vi "Add ECAT Slave.vi"(8 "error in (no error)":errorcluster, 11 "ECAT Master Ref in":T1 format="%.0x") -> (0 "error out":errorcluster, 3 "ECAT Master Ref out":T1 format="%.0x")   [LabVIEW 2016, in "Scan Engine Custom Device.lvlib"]
uses:
  Scan Engine Custom Device.lvlib
  <vilib>/NI Veristand/Custom Device API/Custom Device API.lvlib
  Globals/Scan Engine GUIDs.vi
  Globals/Property Strings.vi
  Type Defs/NI ECAT Slaves.ctl
  <vilib>/NI Veristand/Custom Device API/Custom Device Item Ref.ctl
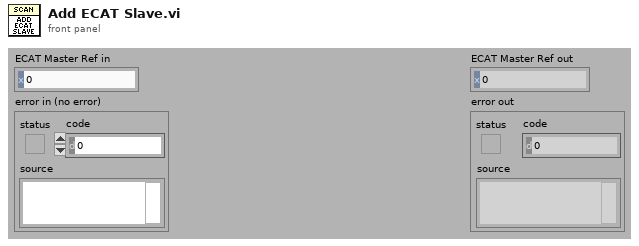
[diagram p1: front panel]
types:
  T1 = typedef "Custom Device API.lvlib/Custom Device Item Ref.ctl" = u64
  T2 = typedef "Scan Engine Custom Device.lvlib/NI ECAT Slaves.ctl" = enum16{"Default", "NI 9144"}
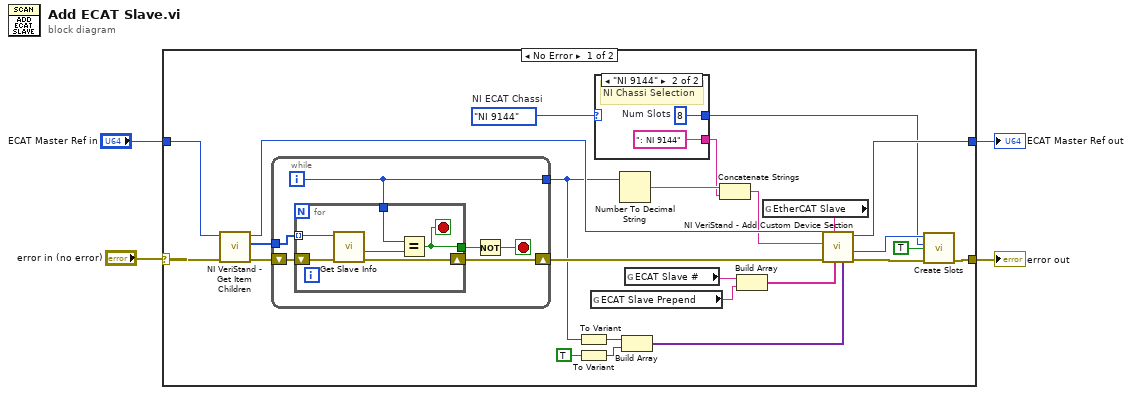
[diagram p0: block diagram]
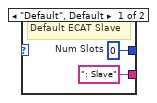
[diagram p2: hidden frame]
diagram:
  n1 = case shown="No Error" "error in (no error)" {
    selector: "error in (no error)" -> [w29 w47]
    tunnel: [w16 w47] -> w3
    tunnel: "ECAT Master Ref in" -> [w28 w46]
    tunnel: [w14 w46] -> w1
    frame No Error {
      w5 = NI_ECAT_Slaves."NI 9144"  # NI ECAT Chassi
      n2 = call <vilib>:"NI VeriStand - Get Item Children.vi"("error in (no error)"=w29, "Item Ref in"=w28) -> ("error out"=w27:errorcluster, "Child Refs"=w26:T1[], "Item Ref out"=w23:T1)  [unwired: 6 in, 1 out]
      n3 = while {
        shift-right: [w35] -> w24
        shift-left: w27 -> [w39]
        tunnel: w26 -> [w38]
        tunnel: [w34] -> w12
        i -> [w34]
        stop <- w36 stop-if-true
        n4 = for {
          tunnel: w38 -> [w42] mode=indexing
          shift-right: [w41] -> w35
          shift-left: w39 -> [w43]
          tunnel: w34 -> [w45]
          tunnel: [w44] -> w37
          stop <- w44 stop-if-true
          n5 = call "Get Slave Info.vi"("error in (no error)"=w43, "Item Ref in"=w42) -> ("error out"=w41:errorcluster, "Slave #"=w40:u16)  [unwired: 5 in, 3 out]
          n6 = Equal?(x=w45, y=w40) -> (x = y?=w44:bool)
        }
        n7 = Not(x=w37) -> (.not. x?=w36:bool)
      }
      n8 = To Variant(anything=w12) -> (Variant=w11:variant)
      n9 = To Variant(anything=TRUE) -> (Variant=w10:variant)
      n10 = global read "Property Strings.vi" "ECAT Slave Prepend"() -> (w13:string)
      n11 = case "Case-Struktur" shown="\"NI 9144\"" w5 {
        tunnel: [w31 w33] -> w7
        tunnel: [": Slave" ("string") ": NI 9144" ("string")] -> w6
        frame "Default", Default {
          w31 = 0  # Num Slots
          # "Default ECAT Slave"
        }
        frame "NI 9144" {
          w33 = 8  # Num Slots
          # "NI Chassi Selection"
        }
      }
      n12 = Number To Decimal String(number=w12) -> (decimal integer string=w20:string)  [unwired: 1 in]
      n13 = Build Array(w11, w10) -> (w8:variant[])
      n14 = global read "Property Strings.vi" "ECAT Slave #"() -> (w22:string)
      n15 = Concatenate Strings(w20, w6) -> (w19:string)
      n16 = Build Array(w22, w13) -> (w21:string[])
      n17 = global read "Scan Engine GUIDs.vi" "EtherCAT Slave"() -> (w25:string)
      n18 = call <vilib>:"NI VeriStand - Add Custom Device Section.vi"("Property Values"=w8, "Property names"=w21, "GUID (Default Section)"=w25, "error in (no error)"=w24, "Section Name"=w19, "Parent Ref in"=w23) -> ("error out"=w17:errorcluster, "Section Ptr"=w15:T1, "Parent Ref out"=w14:T1)  [unwired: 2 in, 1 out]
      n19 = call "Create Slots.vi"("error in"=w17, "EtherCAT?"=TRUE, "Num Slots"=w7, "Item Ref In"=w15) -> ("error out"=w16:errorcluster)  [unwired: 5 in, 1 out]
    }
    frame Error {
    }
  }
  "ECAT Master Ref out" <- w1
  "error out" <- w3
